vi "sutter_test.vi"() -> ()   [LabVIEW 2016]
uses:
  <vilib>/Instr/_visa.llb/VISA Configure Serial Port (Instr).vi
panel:
  in  "Manipulator":u16(ring) items=["DriveA"=1, "DriveB"=2]
  in  "Motor Position":dbl[](array[numeric])
  out "Position XYZ":dbl[](array[numeric])
  in  "Ring":u16(ring) items=["Move to work", "Move to home", "Calibration", "Get pos", "Interrupt", "Move to pos", "ChangeDrive"]
  in  "error in (no error)":errorcluster
  out "error out":errorcluster
  in  "VISA resource name":refnum<visa-resource-name>
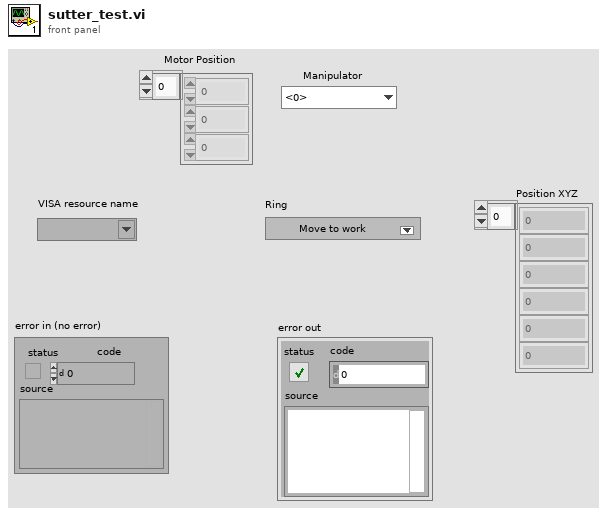
[diagram p1: front panel]
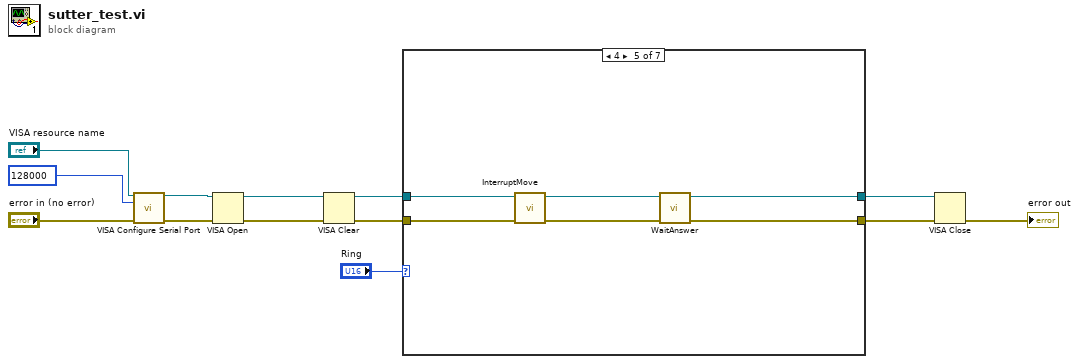
[diagram p0: block diagram]
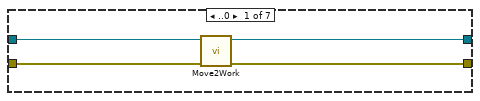
[diagram p2: hidden frame]
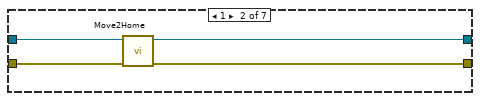
[diagram p3: hidden frame]
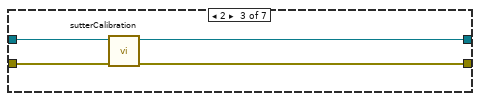
[diagram p4: hidden frame]
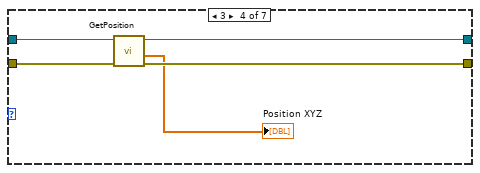
[diagram p5: hidden frame]
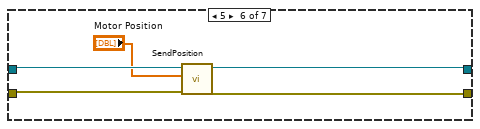
[diagram p6: hidden frame]
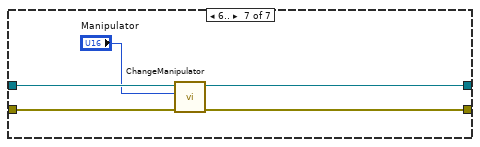
[diagram p7: hidden frame]
diagram:
  n1 = call-poly "VISA Configure Serial Port"("VISA resource name"="VISA resource name", "baud rate (9600)"=u32 128000, "error in (no error)"="error in (no error)") -> ("VISA resource name out"=w10:refnum<visa-resource-name>, "error out"=w8:errorcluster)  [unwired: 11 in]
  n2 = VISA Open(error in (no error)=w8, VISA resource name=w10) -> (VISA resource name=w3:refnum<visa-resource-name>, error out=w4:errorcluster)  [unwired: 3 in]
  n3 = VISA Clear(VISA resource name=w3, error in (no error)=w4) -> (VISA resource name out=w2:refnum<visa-resource-name>, error out=w1:errorcluster)
  n4 = case shown="4" "Ring" {
    tunnel: w2 -> [w17 w20 w25 w30 w36 w41 w46]
    tunnel: w1 -> [w16 w21 w24 w28 w35 w40 w45]
    tunnel: [w15 w18 w22 w27 w31 w38 w43] -> w7
    tunnel: [w14 w19 w23 w29 w32 w39 w44] -> w6
    frame ..0 {
      n5 = call "Move2Work.vi"("error in"=w16, "VISA resource In"=w17) -> ("error out"=w15:errorcluster, "VISA resource name out"=w14:refnum<visa-resource-name>)  [unwired: 6 in]
    }
    frame 1 {
      n6 = call "Move2Home.vi"("error in"=w21, "VISA resource In"=w20) -> ("error out"=w18:errorcluster, "VISA resource name out"=w19:refnum<visa-resource-name>)  [unwired: 6 in]
    }
    frame 2 {
      n7 = call "sutterCalibration.vi"("error in"=w24, "VISA resource In"=w25) -> ("error out"=w22:errorcluster, "VISA resource name out"=w23:refnum<visa-resource-name>)  [unwired: 6 in]
    }
    frame 3 {
      n8 = call "GetPosition.vi"("error in"=w28, "VISA resource name in"=w30) -> ("error out"=w27:errorcluster, "Position XYZ"=→"Position XYZ":dbl[], "VISA resource name out"=w29:refnum<visa-resource-name>)  [unwired: 3 in, 1 out]
    }
    frame 4 {
      n9 = call "InterruptMove.vi"("error in"=w35, "VISA resource In"=w36) -> ("error out"=w34:errorcluster, "VISA resource name out"=w33:refnum<visa-resource-name>)  [unwired: 6 in]
      n10 = call "WaitAnswer.vi"("error in (no error)"=w34, "VISA resource name in"=w33) -> ("error out"=w31:errorcluster, "VISA resource name out"=w32:refnum<visa-resource-name>)  [unwired: 4 in]
    }
    frame 5 {
      n11 = call "SendPosition.vi"("error in"=w40, "Motor Position"="Motor Position", "VISA resource In"=w41) -> ("error out"=w38:errorcluster, "VISA resource name out"=w39:refnum<visa-resource-name>)  [unwired: 5 in]
    }
    frame 6.. {
      n12 = call "ChangeManipulator.vi"("error in"=w45, "Manipulator"="Manipulator", "VISA resource In"=w46) -> ("error out"=w43:errorcluster, "VISA resource name out"=w44:refnum<visa-resource-name>)  [unwired: 5 in]
    }
  }
  n13 = VISA Close(VISA resource name=w6, error in (no error)=w7) -> (error out=→"error out":errorcluster)
